vi "Pfeiffer Vacuum Turbo General operating information.vi"(8 "error in (no error)":errorcluster, 9 "Parameter":u16(ring) items=["nominal speed [Hz] (default) (315)", "intermediate circut current [A] (310)", "motor voltage [V] (313)", "actual power [W] (316)", "operating hours pump [h] (311)", "operating hours drive [h] (314)", "pump cycles (read only) (319)", "status oil sensor (read only) (301)", "speed switchpoint attained (read only) (302)", "overtemperature drive (read only) (304)", "overtemperature pump (read only) (305)", "target speed attained (read only) (306)", "pump accelerates (read only) (307) ", "controlled by remote (300)", "motor phase current [A] (317)", "acceleration / deceleration [rm/s] (336)", "hardware version controller (354)", "target speed (397)", "acutal speed (398)", "nominal speed (399)", "software version control unit (read only) (352)"], 10 "Adress of unit":u16=1 min=1 max=999 step=1, 11 "COM Port Name in":refnum<visa-resource-name>="COM1") -> (0 "error out":errorcluster, 3 "response (data)":string)   [LabVIEW 2021]
doc: "This VI is an example of how to use the Pfeiffer Vacuum subVIs programmatically. This VI first initializes the instrument, takes measurements, then closes the instrument."
uses:
  <instrlib>/Pfeiffer Vacuum/Pfeiffer Vacuum.lvlib
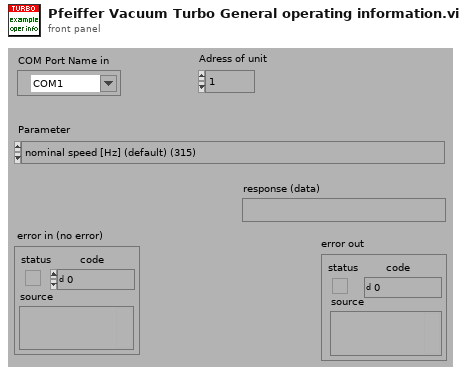
[diagram p1: front panel]
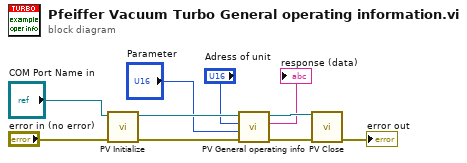
[diagram p0: block diagram]
diagram:
  n1 = call <instrlib>:"PV Initialize.vi"("error in (no error)"="error in (no error)", "VISA session in"="COM Port Name in") -> ("error out"=w10:errorcluster, "VISA session out"=w8:refnum<visa-resource-name>)  [unwired: 8 in]
  n2 = call <instrlib>:"PV General operating info.vi"("error in (no error)"=w10, "Parameter"="Parameter", "Adress of unit"="Adress of unit", "VISA session"=w8) -> ("error out"=w9:errorcluster, "response (data)"=→"response (data)":string, "dup VISA session"=w7:refnum<visa-resource-name>)  [unwired: 5 in]
  n3 = call <instrlib>:"PV Close.vi"("VISA session"=w7, "error in (no error)"=w9) -> ("error out"=→"error out":errorcluster)  [unwired: 13 in]
